vi "Move Control with Keyboard.vi"() -> ()   [LabVIEW 2022 SP3]
uses:
  <vilib>/Utility/miscctls.llb/LVPositionTypeDef.ctl
panel:
  out "Top":bool
  out "exit?":bool
  in  "STOP":bool
  out "BarPosition":T1
  out "BallPosition":T1
  out "Step":T1
  out "Score":i32
  out "Bar":bool
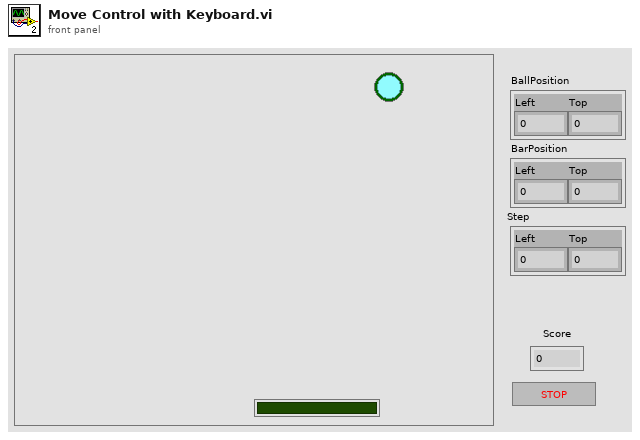
[diagram p1: front panel]
types:
  T1 = typedef "LVPositionTypeDef.ctl" = cluster{"Left":i32, "Top":i32}
  T2 = cluster{"BallPosition":T1, "Step":T1, "Score":i32, "BarPosition":T1}
  T3 = typedef "LVBoundsTypeDef.ctl" = cluster{"Width":u32, "Height":u32}
  T4 = typedef "eventvkey.ctl" = enum16{"ASCII", "Enter", "Return", "Shift", "Ctrl", "Alt", "Cmd", "Opt", "Caps", "NumLock", "Clear", "Break", "Up", "Down", "Left", "Right", "Insert", "Delete", "Home", "End", "PageUp", "PageDown", "Escape", "Help", "Pause", "ScrollLock", "F1", "F2", "F3", "F4", "F5", "F6", "F7", "F8", "F9", "F10", "F11", "F12", "F13", "F14", "F15", "F16", "F17", "F18", "F19", "F20", "F21", "F22", "F23", "F24", "Play", "VolumeUp", "VolumeDown", "Mute", "Two Byte Char"}
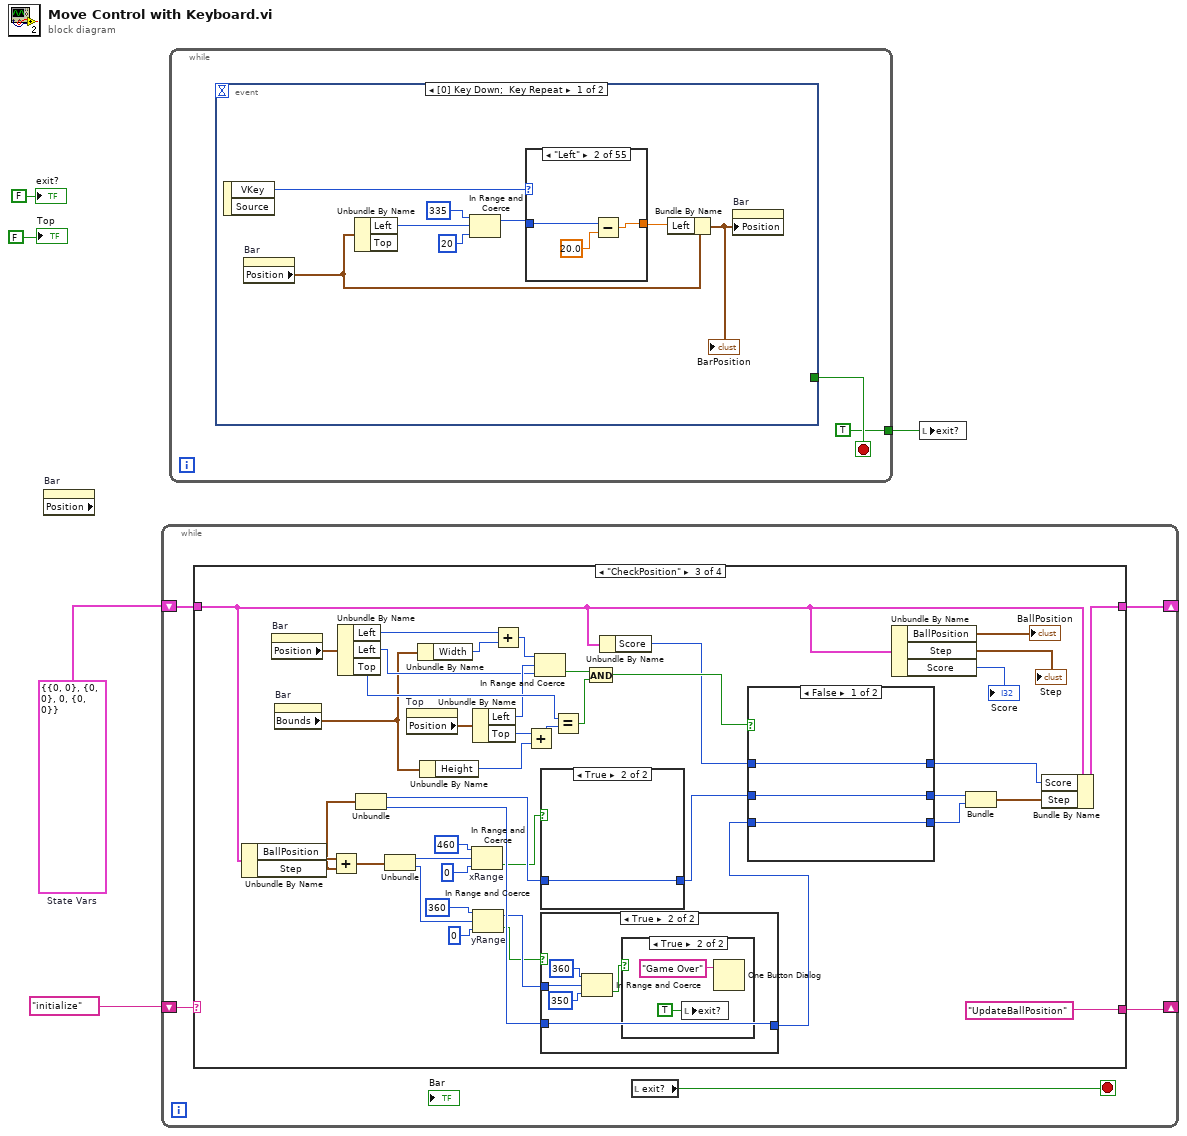
[diagram p0: block diagram]
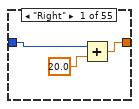
[diagram p2: hidden frame]
diagram:
  w4 = T2 {"BallPosition"={"Left"=0, "Top"=0}, "Step"={"Left"=0, "Top"=0}, "Score"=0, "BarPosition"={"Left"=0, "Top"=0}}  # State Vars
  n1 = property on="Bar" class="Bool (strict)" props=["Position"]() -> ()  [unwired: 2 in, 3 out]
  n2 = while {
    shift-right: [w8] -> _
    shift-left: "initialize" -> [w7]
    shift-right: [w9] -> _
    shift-left: w4 -> [w10]
    stop <- w6 stop-if-true
    n3 = case shown="\"CheckPosition\"" w7 {
      selector: w7 -> [w11 _ _ _]
      tunnel: w10 -> [w12 w18 w30 w81]
      tunnel: [w12 w17 w50 w85] -> w9
      tunnel: [w11 "UpdateBallPosition" "UpdateBallPosition" "CheckPosition"] -> w8
      frame "False", Default {
      }
      frame "Initialize" {
        n4 = Bundle By Name(cluster=w18, "BallPosition"=T1 {"Left"=240, "Top"=180} ("Position"), "Step"=T1 {"Left"=1, "Top"=1}, "BarPosition"=T1 {"Left"=0, "Top"=0}) -> (w17:T2)
      }
      frame "CheckPosition" {
        n5 = Unbundle By Name(w30) -> ("BallPosition"=w60:T1, "Step"=w39:T1)
        n6 = property on="Bar" class="Bool (strict)"() -> ("Position"=w43:T1)  [unwired: 2 in, 2 out]
        n7 = property on="Bar" class="Bool (strict)"() -> ("Bounds"=w20:T3)  [unwired: 2 in, 2 out]
        n8 = Add(x=w60, y=w39) -> (x+y=w59:T1)
        n9 = Unbundle By Name(w43) -> ("Left"=w44:i32, "Left"=w24:i32, "Top"=w26:i32)
        n10 = Unbundle(w39) -> ("Left"=w52:i32, "Top"=w51:i32)
        n11 = Unbundle(w59) -> ("Left"=w58:i32, "Top"=w53:i32)
        n12 = property on="Top" class="Bool (strict)"() -> ("Position"=w42:T1)  [unwired: 2 in, 2 out]
        n13 = Unbundle By Name(w20) -> ("Width"=w21:u32)
        n14 = Unbundle By Name(w20) -> ("Height"=w19:u32)
        n15 = In Range and Coerce "xRange"(upper limit=460, x=w58, lower limit=0) -> (In Range?=w41:bool)  [unwired: 1 out]
        n16 = Unbundle By Name(w42) -> ("Left"=w25:i32, "Top"=w23:i32)
        n17 = In Range and Coerce "yRange"(upper limit=360, x=w53, lower limit=0) -> (coerced(x)=w48:i32, In Range?=w40:bool)
        n18 = Add(x=w44, y=w21) -> (x+y=w45:u32)
        n19 = Add(x=w23, y=w19) -> (x+y=w22:u32)
        n20 = In Range and Coerce(upper limit=w45, x=w25, lower limit=w24) -> (In Range?=w47:bool)  [unwired: 1 out]
        n21 = case shown="True" w41 {
          tunnel: [w78 w80] -> w37
          tunnel: w52 -> [w79 w80]
          frame False {
            n22 = Negate(x=w79) -> (-x=w78:i32)
          }
          frame True {
          }
        }
        n23 = case shown="True" w40 {
          tunnel: [w70 w75] -> w38
          tunnel: w51 -> [w69 w75]
          tunnel: w48 -> [_ w72]
          frame False {
            n24 = Negate(x=w69) -> (-x=w70:i32)
          }
          frame True {
            n25 = In Range and Coerce(upper limit=360, x=w72, lower limit=350) -> (In Range?=w71:bool)  [unwired: 1 out]
            n26 = case shown="True" w71 {
              frame False {
              }
              frame True {
                n27 = local write "exit?"(TRUE ("exit?")) -> ()
                n28 = One Button Dialog(message="Game Over") -> ()  [unwired: 1 in, 1 out]
              }
            }
          }
        }
        n29 = Equal?(x=w26, y=w22) -> (x = y?=w46:bool)
        n30 = And(x=w47, y=w46) -> (x .and. y?=w33:bool)
        n31 = Unbundle By Name(w30) -> ("Score"=w32:i32)
        n32 = case shown="False" w33 {
          tunnel: w38 -> [w62 w68]
          tunnel: w37 -> [w63 w64]
          tunnel: [w63 w64] -> w35
          tunnel: [w62 w67] -> w36
          tunnel: w32 -> [w61 w66]
          tunnel: [w61 w65] -> w31
          frame False {
          }
          frame True {
            n33 = Negate(x=w68) -> (-x=w67:i32)
            n34 = Increment(x=w66) -> (x+1=w65:i32)
          }
        }
        n35 = Unbundle By Name(w30) -> ("BallPosition"=→"BallPosition":T1, "Step"=→"Step":T1, "Score"=→"Score":i32)
        n36 = Bundle("Left"=w35, "Top"=w36) -> (w34:cluster{"Left":i32, "Top":i32})  [unwired: 1 in]
        n37 = Bundle By Name(cluster=w30, "Score"=w31, "Step"=w34) -> (w50:T2)
      }
      frame "UpdateBallPosition" {
        n38 = Unbundle By Name(w81) -> ("BallPosition"=w86:T1, "Step"=w87:T1)
        n39 = Add(x=w86, y=w87) -> (x+y=w84:T1)
        n40 = Bundle By Name(cluster=w81, "BallPosition"=w84) -> (w85:T2)
        n41 = property on="Top" class="Bool (strict)"("Position"=w84) -> ()  [unwired: 2 in, 2 out]
        n42 = Wait (ms)(milliseconds to wait=u32 7) -> ()  [unwired: 1 out]
      }
    }
    n43 = local read "exit?"() -> (w6:bool)
  }
  n44 = while {
    tunnel: [TRUE ("Top")] -> w1
    stop <- w89 stop-if-true
    n45 = event shown="[0] Key Down;  Key Repeat" {
      selector: _ -> [_ _]
      dyn-events: _ -> [_ _]
      timeout: _ -> [_ _]
      tunnel: [_ "STOP"] -> w89
      event Key Down; Key Repeat {
        n46 = event-data() -> ("VKey"=w90:T4)  [unwired: 1 in, 1 out]
        n47 = property on="Bar" class="Bool (strict)"() -> ("Position"=w96:T1)  [unwired: 2 in, 2 out]
        n48 = Unbundle By Name(w96) -> ("Left"=w93:i32)  [unwired: 1 out]
        n49 = In Range and Coerce(upper limit=335, x=w93, lower limit=20) -> (coerced(x)=w94:i32)  [unwired: 1 out]
        n50 = case shown="\"Left\"" w90 {
          tunnel: w94 -> [w99 w101 w104 w105 w106 w107 w108 w109 w110 w111 w112 w113 w114 w115 w116 w117 w118 w119 w120 w121 w122 w123 w124 w125 w126 w127 w128 w129 w130 w131 w132 w133 w134 w135 w136 w137 w138 w139 w140 w141 w142 w143 w144 w145 w146 w147 w148 w149 w150 w151 w152 w153 w154 w155 w156]
          tunnel: [w98 w102 w104 w105 w106 w107 w108 w109 w110 w111 w112 w113 w114 w115 w116 w117 w118 w119 w120 w121 w122 w123 w124 w125 w126 w127 w128 w129 w130 w131 w132 w133 w134 w135 w136 w137 w138 w139 w140 w141 w142 w143 w144 w145 w146 w147 w148 w149 w150 w151 w152 w153 w154 w155 w156] -> w97
          frame "Right" {
            n51 = Add(x=w99, y=20.0) -> (x+y=w98:dbl)
          }
          frame "Left" {
            n52 = Subtract(x=w101, y=20.0) -> (x-y=w102:dbl)
          }
          frame "F16" {
          }
          frame "F17" {
          }
          frame "F18" {
          }
          frame "F19" {
          }
          frame "F20" {
          }
          frame "F21" {
          }
          frame "F22" {
          }
          frame "F23" {
          }
          frame "F24" {
          }
          frame "Play" {
          }
          frame "VolumeUp" {
          }
          frame "VolumeDown" {
          }
          frame "Mute" {
          }
          frame "Two Byte Char" {
          }
          frame "Insert" {
          }
          frame "Delete" {
          }
          frame "Home" {
          }
          frame "End" {
          }
          frame "PageUp" {
          }
          frame "PageDown" {
          }
          frame "Escape" {
          }
          frame "Help" {
          }
          frame "Pause" {
          }
          frame "ScrollLock" {
          }
          frame "F1" {
          }
          frame "F2" {
          }
          frame "F3" {
          }
          frame "F4" {
          }
          frame "F5" {
          }
          frame "F6" {
          }
          frame "F7" {
          }
          frame "F8" {
          }
          frame "F9" {
          }
          frame "F10" {
          }
          frame "F11" {
          }
          frame "F12" {
          }
          frame "F13" {
          }
          frame "F14" {
          }
          frame "F15" {
          }
          frame "Down" {
          }
          frame "Up" {
          }
          frame "Break" {
          }
          frame "Clear" {
          }
          frame "NumLock" {
          }
          frame "Caps" {
          }
          frame "Opt" {
          }
          frame "Cmd" {
          }
          frame "Alt" {
          }
          frame "Ctrl" {
          }
          frame "Shift" {
          }
          frame "Return" {
          }
          frame "Enter" {
          }
          frame "ASCII" {
          }
        }
        n53 = Bundle By Name(cluster=w96, "Left"=w97) -> (w95:T1)
        "BarPosition" <- w95
        n54 = property on="Bar" class="Bool (strict)"("Position"=w95) -> ()  [unwired: 2 in, 2 out]
      }
      event "STOP": Value Change {
        n55 = event-data() -> ()  [unwired: 1 in, 4 out]
      }
    }
  }
  n56 = local write "exit?"(w1) -> ()
  "exit?" <- FALSE ("exit?")
  "Top" <- FALSE ("Top")
